vi "SSC DCPower Get SMU Models.vi"(0 "DCPower SSC in":T1[](array[typedef]), 11 "error in":errorcluster) -> (4 "DCPower SSC out":T1[](array[typedef]), 6 "SMU Models":string[](array[string]), 15 "error out":errorcluster)   [LabVIEW 2019]
doc: "This VI gets the 4-digit numerical model number for each DCPower Session.\n\nFor example, this will return \"4139\" for a PXIe-4139 SMU."
uses:
  SSC DCPower.ctl
  <vilib>/regexp/Match Regular Expression.xnode
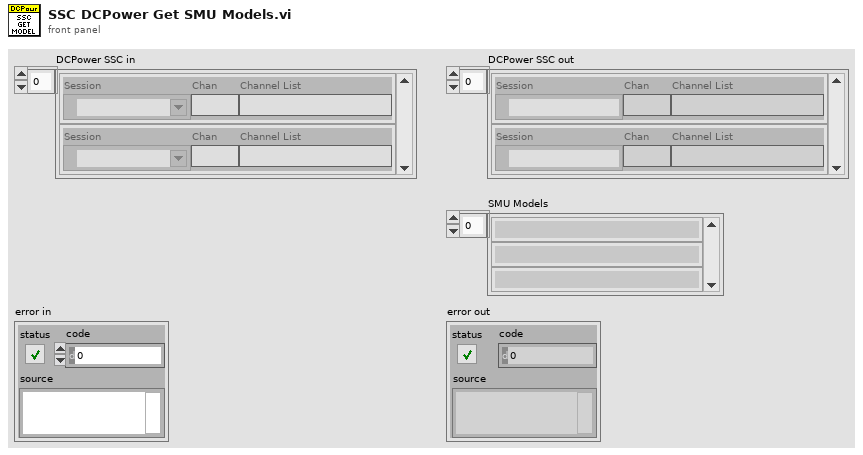
[diagram p1: front panel]
types:
  T1 = typedef "SSC DCPower.ctl" = cluster{"Session":refnum<k15>, "Chan":string, "Channel List":string}
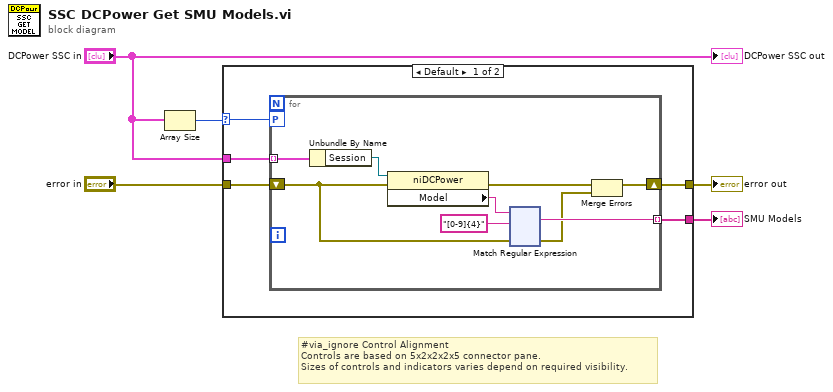
[diagram p0: block diagram]
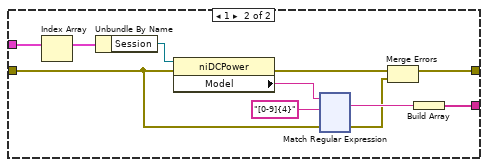
[diagram p2: hidden frame]
diagram:
  # "#via_ignore Control Alignment\nControls are based on 5x2x2x2x5 connector pane.\nSizes of controls and indicators varies depend on required visibility."
  n1 = Array Size(array="DCPower SSC in") -> (size(s)=w1:i32)
  n2 = case shown="Default" w1 {
    selector: w1 -> [w6 _]
    tunnel: "DCPower SSC in" -> [w10 w144]
    tunnel: "error in" -> [w9 w136]
    tunnel: [w8 w135] -> w4
    tunnel: [w7 w138] -> w3
    frame Default {
      n3 = for {
        tunnel: w10 -> [w19] mode=indexing
        shift-right: [w12] -> w8
        shift-left: w9 -> [w13]
        tunnel: [w14] -> w7 mode=indexing
        workers-P: w6 -> [_]
        n4 = Unbundle By Name(w19) -> ("Session"=w18:refnum<k15>)
        n5 = property class="niDCPower"(reference=w18, error in=w13) -> (error out=w17:errorcluster, "Model"=w16:string)  [unwired: 1 out]
        n6 = xnode "Match Regular Expression"("input string"=w16, "regular expression"="[0-9]{4}", "error in"=w13) -> ("whole match"=w14:string, "error out"=w11:errorcluster)  [unwired: 3 in, 3 out]
        n7 = Merge Errors(w17, w11) -> (w12:errorcluster)
      }
    }
    frame 1 {
      n8 = Index Array(array=w144) -> (element=w137:T1)  [unwired: 1 in]
      n9 = Unbundle By Name(w137) -> ("Session"=w141:refnum<k15>)
      n10 = property class="niDCPower"(reference=w141, error in=w136) -> (error out=w143:errorcluster, "Model"=w140:string)  [unwired: 1 out]
      n11 = xnode "Match Regular Expression"("input string"=w140, "regular expression"="[0-9]{4}", "error in"=w136) -> ("whole match"=w142:string, "error out"=w134:errorcluster)  [unwired: 3 in, 3 out]
      n12 = Merge Errors(w143, w134) -> (w135:errorcluster)
      n13 = Build Array(w142) -> (w138:string[])
    }
  }
  "error out" <- w4
  "SMU Models" <- w3
  "DCPower SSC out" <- "DCPower SSC in"
